vi "Send-heartbeat.vi"(8 "error in (no error)":errorcluster, 11 "Client in":T1) -> (0 "error out":errorcluster, 3 "Client out":T1)   [LabVIEW 2013, in "Client.lvlib" / "Client.lvclass"]
doc: "Wrapper function for sending the specific 'Hearbeat' type message.\nThis function creates and immediately sends a heartbeat message to the server, using the configuration of the client object."
uses:
  Client.lvclass
  Object-reference.ctl
  Client.lvclass/Client.ctl
  Messages/Sources/Heartbeat/Heartbeat.lvclass
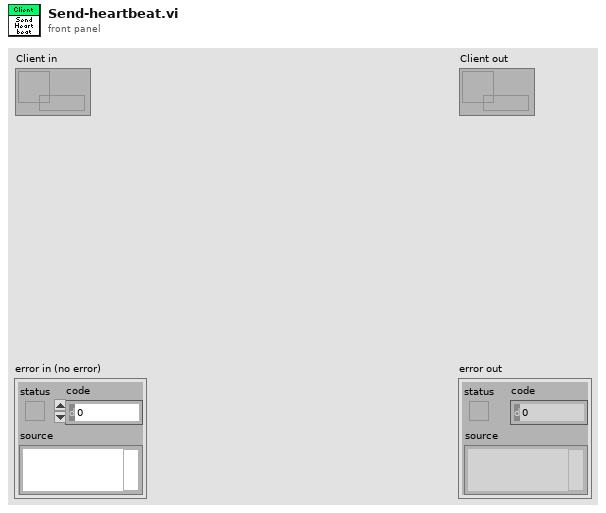
[diagram p1: front panel]
types:
  T1 = typedef "Client.lvlib/Client.lvclass/Object-reference.ctl" = refnum<data-value>
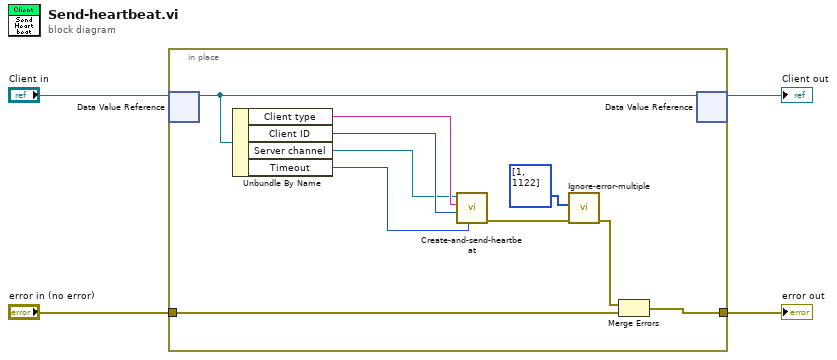
[diagram p0: block diagram]
diagram:
  n1 = in-place {
    in-place-border: "error in (no error)" -> [w5]
    in-place-border: [w6] -> w3
    n2 = in-place-dvr #1("Client in") -> (w9:refnum<class "Client.lvclass">)  [unwired: 1 out]
    n3 = Unbundle By Name(w9) -> ("Client type"=w14:string, "Client ID"=w13:i32, "Server channel"=w12:refnum<queue>, "Timeout"=w11:i32)
    n4 = call "Create-and-send-heartbeat.vi"("Timeout"=w11, "Sender ID"=w13, "Sender"=w14, "Server channel"=w12) -> ("error out"=w10:errorcluster)  [unwired: 7 in]
    n5 = call "Ignore-error-multiple.vi"("error in (no error)"=w10, "Errors to ignore (1)"=i32[] [1, 1122]) -> ("error out"=w8:errorcluster)  [unwired: 9 in]
    n6 = Merge Errors(w8, w5) -> (w6:errorcluster)
    n7 = in-place-dvr #1(w9) -> (→"Client out":T1)  [unwired: 1 out]
  }
  "error out" <- w3
